vi "Untitled 5.vi"() -> ()   [LabVIEW 2018]
uses:
  <vilib>/Utility/file.llb/Read Delimited Spreadsheet (string).vi
  <vilib>/Utility/file.llb/Read Delimited Spreadsheet (DBL).vi
panel:
  in  "file path (dialog if empty)":path
  out "Array 4":bool[](array[boolean])
  in  "Array 3":bool[](array[boolean])
  in  "Array 2":dbl[](array[slide]) scale=0.0..10.0
  out "Array":dbl[](array[numeric])
  out "Table Control":string[][](table)
  out "Waveform Graph":dbl[][](graph)
  in  "Path":path
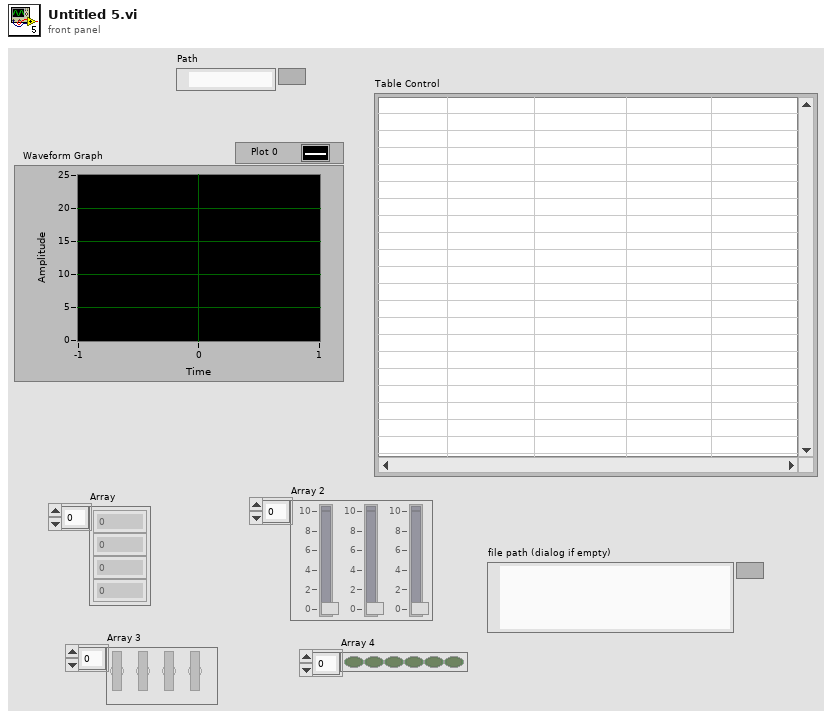
[diagram p1: front panel]
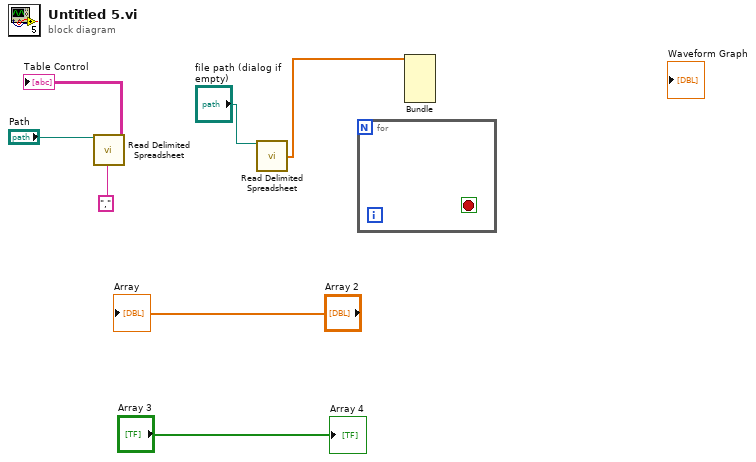
[diagram p0: block diagram]
diagram:
  n1 = call-poly <vilib>:"Read Delimited Spreadsheet.vi"("file path (dialog if empty)"="Path", "delimiter (\\t)"=",") -> ("all rows"=→"Table Control":string[][])  [unwired: 8 in, 5 out]
  n2 = call-poly <vilib>:"Read Delimited Spreadsheet.vi"("file path (dialog if empty)"="file path (dialog if empty)") -> ("first row"=w1:dbl[])  [unwired: 9 in, 5 out]
  n3 = for {
    stop <- _ stop-if-true
  }
  n4 = Bundle("first row"=w1) -> ()  [unwired: 6 in, 1 out]
  "Array" <- "Array 2"
  "Array 4" <- "Array 3"
